vi "qc5psm2.vi"() -> ()   [LabVIEW 2020]
uses:
  <instrlib>/CAEN PSM/CAEN PSM.lvlib
panel:
  in  "Tab Control":enum32{"Page 1"}(tab)
  in  "Tab Control 2":enum32{"Page 1", "Page 2"}(tab)
  out "RDW":bool
  out "V monitor":dbl(graph)
  out "I monitor":dbl(graph)
  out "SHUT DOWN":bool
  out "COUNT VALUE":dynamicdata(graph)
  in  "count Time(sec)":dbl=60.0
  in  "Final Voltage":dbl=3250.0
  in  "V_step 1":dbl=200.0
  in  "VISA resource name":refnum<visa-resource-name>
  in  "Voltage ramp up (0 V/s)":u16 max=999
  in  "Voltage Max (0.0 V)":u16 max=9999
  in  "Board Address":i8 max=31
  in  "Vset_initial":dbl=100.0
  out "OVV 2":bool
  out "OVC 2":bool
  out "R calc":dbl
  out "Actual current level (Imon)":dbl
  out "Actual voltage level (Vmon)":dbl
  in  "START AGAIN":bool
  out "Channel Status Array":T1(array[cluster])
  in  "Channel (0)":u8=1
  in  "Req (Mohm)":dbl
  out "I set status":dbl
  in  "stop":bool
  in  "Middle Volt":dbl=3000.0
  in  "V step 2":dbl=100.0
  out "COUNT ON  TIMES":i16
  in  "device name":tag="Dev1"
  out "Counts":dbl
  out "time eclapsed":dbl format="%<%H:%M>t"
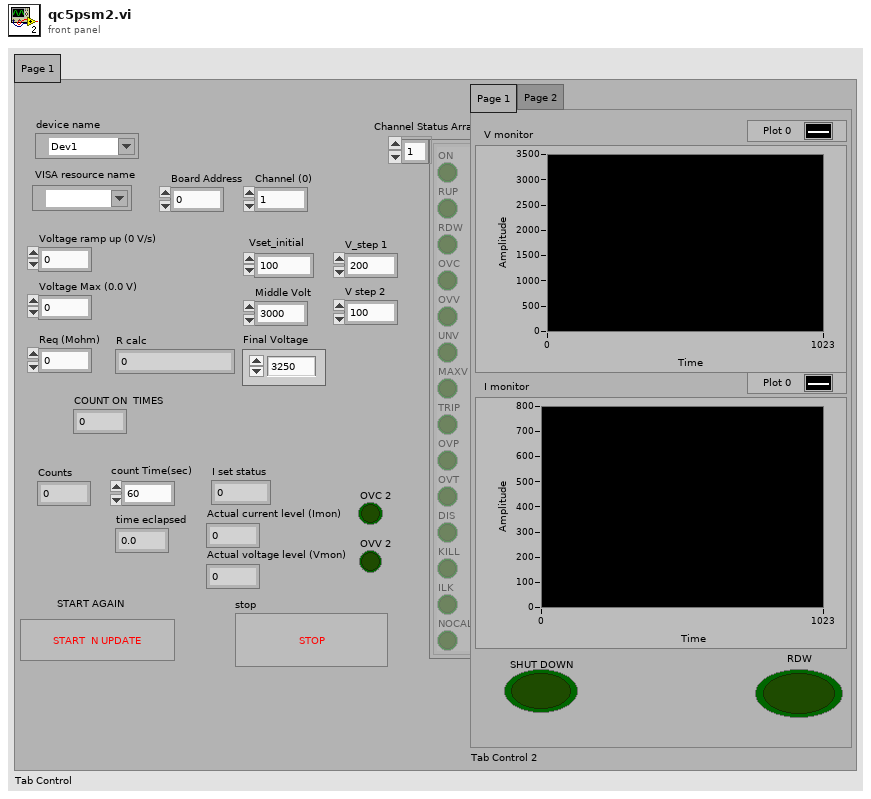
[diagram p1: front panel]
types:
  T1 = cluster{"ON":bool, "RUP":bool, "RDW":bool, "OVC":bool, "OVV":bool, "UNV":bool, "MAXV":bool, "TRIP":bool, "OVP":bool, "OVT":bool, "DIS":bool, "KILL":bool, "ILK":bool, "NOCAL":bool}[]
  T2 = cluster{"Baud Rate":u32, "Parity":enum16{"None", "Odd", "Even", "Mark", "Space"}, "Data Bits":u16, "Stop Bits":u16, "Flow Control":u16}
  T3 = typedef "CAEN PSM.lvlib/BoardHandle.ctl" = cluster{"VISA resource name":refnum<visa-resource-name>, "Board address":i8, "NChannels":u8}
  T4 = cluster{"ON":bool, "RUP":bool, "RDW":bool, "OVC":bool, "OVV":bool, "UNV":bool, "MAXV":bool, "TRIP":bool, "OVP":bool, "OVT":bool, "DIS":bool, "KILL":bool, "ILK":bool, "NOCAL":bool}
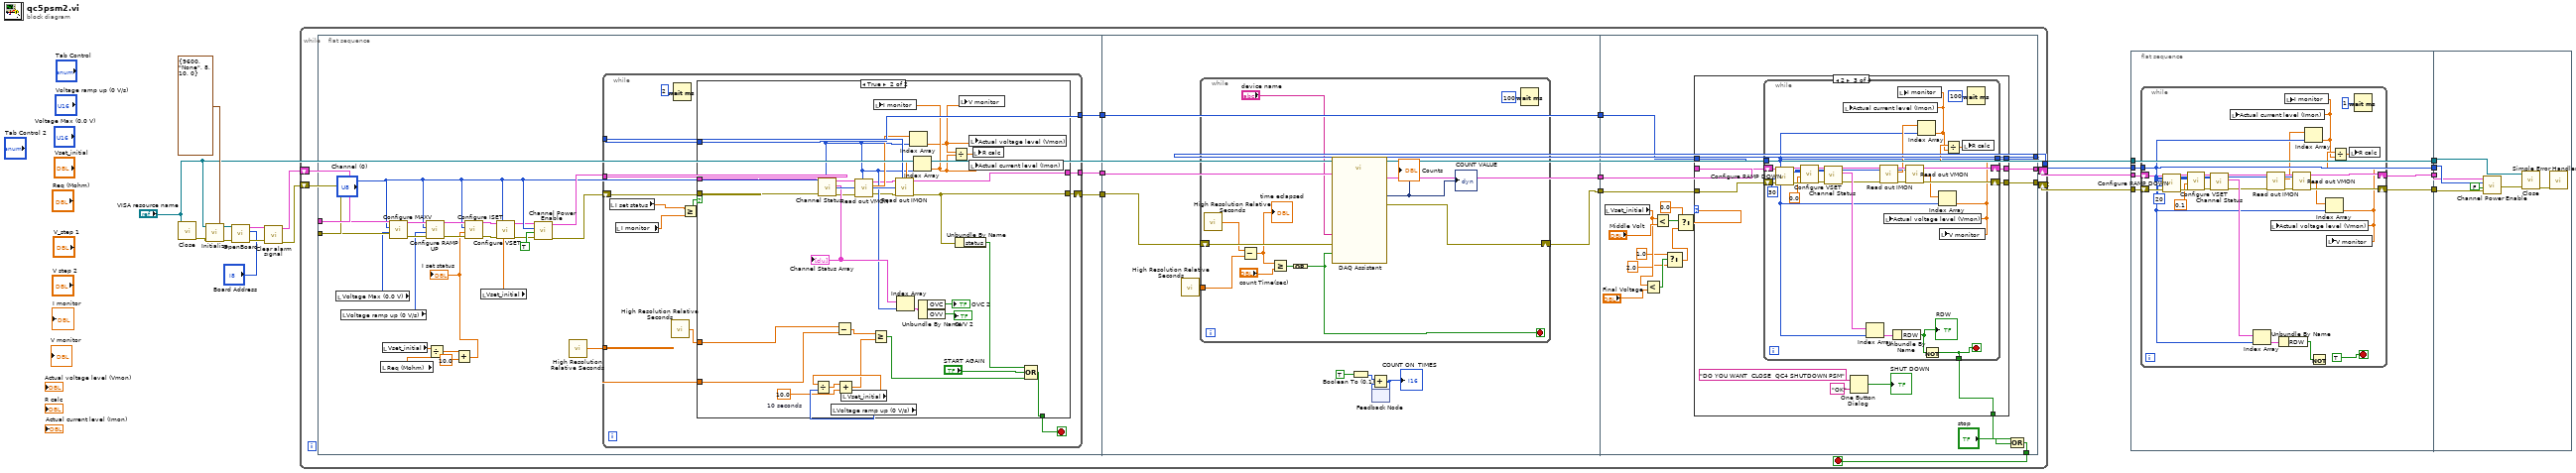
[diagram p0: block diagram]
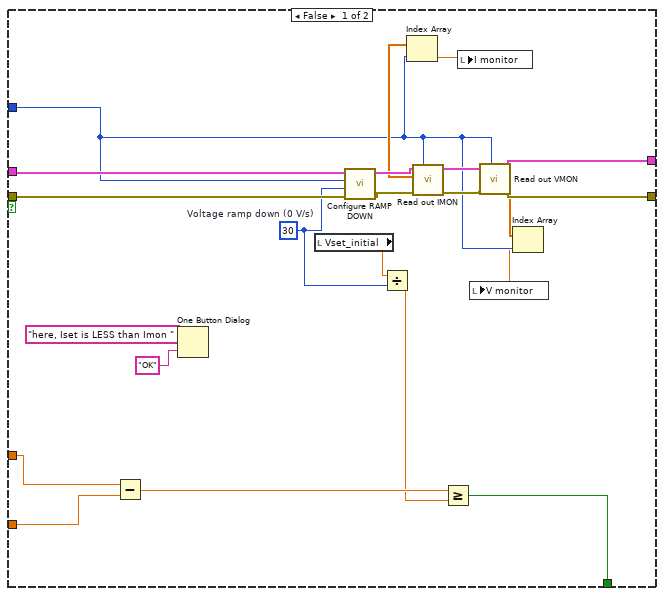
[diagram p2: hidden frame]
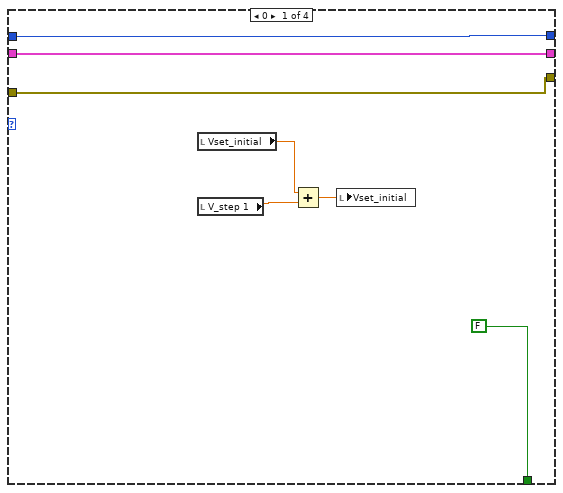
[diagram p3: hidden frame]
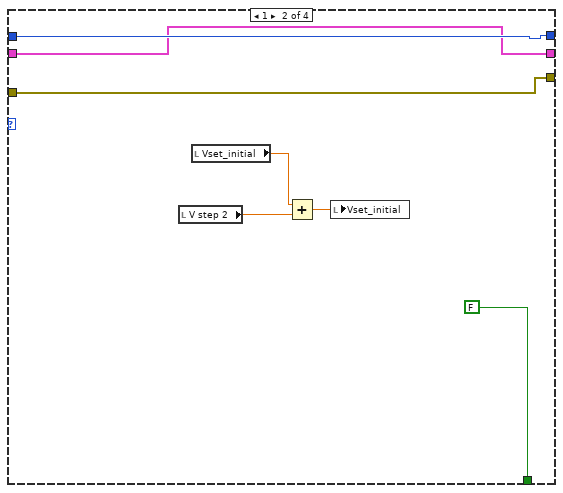
[diagram p4: hidden frame]
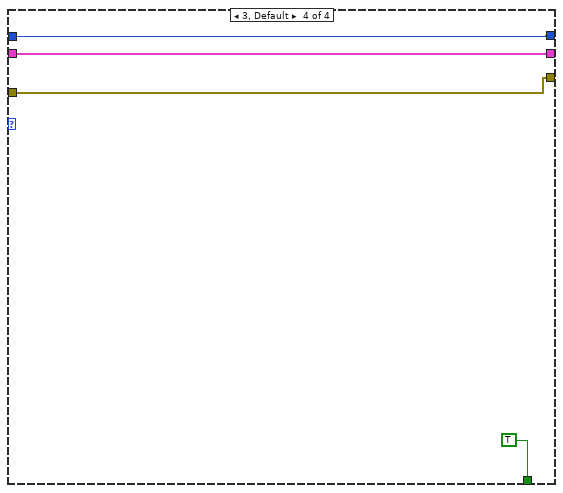
[diagram p5: hidden frame]
diagram:
  n1 = call <instrlib>:"Close.vi"("VISA resource name"="VISA resource name") -> ("error out"=w8:errorcluster)  [unwired: 10 in]
  n2 = call <instrlib>:"Initialize.vi"("Serial Configuration"=T2 {"Baud Rate"=9600, "Parity"=enum."None", "Data Bits"=8, "Stop Bits"=10, "Flow Control"=0}, "error in (no error)"=w8, "VISA resource name"="VISA resource name") -> ("error out"=w7:errorcluster, "VISA resource name out"=w16:refnum<visa-resource-name>)  [unwired: 7 in]
  n3 = call <instrlib>:"OpenBoard.vi"("error in (no error)"=w7, "Board Address"="Board Address", "VISA resource name"=w16) -> ("error out"=w14:errorcluster, "BoardHandle"=w15:T3)  [unwired: 7 in]
  n4 = call <instrlib>:"Clear alarm signal.vi"("error in (no error)"=w14, "BoardHandle"=w15) -> ("error out"=w9:errorcluster, "BoardHandle out"=w10:T3)  [unwired: 8 in]
  n5 = while {
    tunnel: [w29] -> w11
    shift-right: [w26] -> w6
    shift-left: w10 -> [w28]
    shift-right: [w18] -> w5
    shift-left: w9 -> [w27]
    stop <- w25 stop-if-true
    n6 = flat-sequence {
      tunnel: w28 -> [w53]
      tunnel: w27 -> [w52]
      tunnel: [w54] -> w24
      tunnel: [w33] -> w22
      tunnel: [w32] -> w20
      tunnel: w24 -> [w128]
      tunnel: [w128] -> w23
      tunnel: w22 -> [w127]
      tunnel: [w127] -> w21
      tunnel: w20 -> [w126]
      tunnel: [w125] -> w19
      tunnel: [w141] -> w18
      tunnel: [w140] -> w26
      tunnel: [w144] -> w29
      tunnel: w23 -> [w145]
      tunnel: w21 -> [w143]
      tunnel: w19 -> [w142]
      tunnel: [w147] -> w25
      frame #0 {
        n7 = local read "Voltage Max (0.0 V)"() -> (w48:u16)
        n8 = local read "Voltage ramp up (0 V/s)"() -> (w47:u16)
        n9 = local read "Req (Mohm)"() -> (w37:dbl)
        n10 = local read "Vset_initial"() -> (w38:dbl)
        n11 = call <instrlib>:"Configure MAXV.vi"("error in (no error)"=w52, "Voltage Max (0.0 V)"=w48, "Channel (0)"="Channel (0)", "BoardHandle"=w53) -> ("error out"=w49:errorcluster, "BoardHandle out"=w50:T3)  [unwired: 6 in]
        n12 = call <instrlib>:"Configure RAMP UP.vi"("error in (no error)"=w49, "Voltage ramp up (0 V/s)"=w47, "Channel (0)"="Channel (0)", "BoardHandle"=w50) -> ("error out"=w43:errorcluster, "BoardHandle out"=w45:T3)  [unwired: 6 in]
        n13 = Divide(x=w38, y=w37) -> (x/y=w40:dbl)
        n14 = Add(x=w40, y=10.0) -> (x+y=w30:dbl)
        "I set status" <- w30
        n15 = call <instrlib>:"Configure ISET.vi"("error in (no error)"=w43, "Current Limit (0.00 uA)"=w30, "Channel (0)"="Channel (0)", "BoardHandle"=w45) -> ("error out"=w42:errorcluster, "BoardHandle out"=w44:T3)  [unwired: 6 in]
        n16 = local read "Vset_initial"() -> (w41:dbl)
        n17 = call <instrlib>:"Configure VSET.vi"("error in (no error)"=w42, "Voltage Level (0.0 V)"=w41, "Channel (0)"="Channel (0)", "BoardHandle"=w44) -> ("error out"=w35:errorcluster, "BoardHandle out"=w34:T3)  [unwired: 6 in]
        n18 = call <instrlib>:"Channel Power Enable.vi"("error in (no error)"=w35, "Enable (OFF)"=TRUE, "Channel (0)"="Channel (0)", "BoardHandle"=w34) -> ("error out"=w51:errorcluster, "BoardHandle out"=w55:T3)  [unwired: 6 in]
        n19 = call <vilib>:"High Resolution Relative Seconds.vi"() -> ("relative seconds"=w31:dbl)
        n20 = while {
          shift-right: [w63] -> w32
          shift-left: w51 -> [w64]
          tunnel: [w62] -> w33
          tunnel: [w67] -> w54
          tunnel: w55 -> [w65]
          tunnel: "Channel (0)" -> [w67]
          tunnel: w31 -> [w60]
          stop <- w59 stop-if-true
          n21 = local read "I set status"() -> (w58:dbl)
          n22 = local read "I monitor"() -> (w56:dbl)
          n23 = call <vilib>:"High Resolution Relative Seconds.vi"() -> ("relative seconds"=w57:dbl)
          n24 = Wait (ms)(milliseconds to wait=u32 2) -> ()  [unwired: 1 out]
          n25 = Greater Or Equal?(x=w58, y=w56) -> (x >= y?=w61:bool)
          n26 = case shown="True" w61 {
            tunnel: w67 -> [w73 w113]
            tunnel: w65 -> [w89 w112]
            tunnel: w64 -> [w88 w111]
            tunnel: [w76 w110] -> w63
            tunnel: [w77 w109] -> w62
            tunnel: w60 -> [w87 w104]
            tunnel: [w82 w99] -> w59
            tunnel: w57 -> [w68 w90]
            frame False {
              w84 = u16 30  # Voltage ramp down (0 V/s)
              n27 = Subtract(x=w68, y=w87) -> (x-y=w86:dbl)
              n28 = One Button Dialog(message="here, Iset is LESS than Imon ", button name ("OK")="OK") -> ()  [unwired: 1 out]
              n29 = local read "Vset_initial"() -> (w85:dbl)
              n30 = call <instrlib>:"Configure RAMP DOWN.vi"("error in (no error)"=w88, "Voltage ramp down (0 V/s)"=w84, "Channel (0)"=w73, "BoardHandle"=w89) -> ("error out"=w80:errorcluster, "BoardHandle out"=w81:T3)  [unwired: 6 in]
              n31 = Divide(x=w85, y=w84) -> (x/y=w83:dbl)
              n32 = call <instrlib>:"Read out IMON.vi"("Channel"=w73, "error in (no error)"=w80, "BoardHandle"=w81) -> ("error out"=w78:errorcluster, "IMon values (uA)"=w75:dbl[], "BoardHandle out"=w79:T3)  [unwired: 5 in, 1 out]
              n33 = Index Array(array=w75, index=w73) -> (element=w70:dbl)
              n34 = Greater Or Equal?(x=w86, y=w83) -> (x >= y?=w82:bool)
              n35 = local write "I monitor"(w70) -> ()
              n36 = call <instrlib>:"Read out VMON.vi"("Channel"=w73, "error in (no error)"=w78, "BoardHandle"=w79) -> ("error out"=w76:errorcluster, "VMon values (V)"=w74:dbl[], "BoardHandle out"=w77:T3)  [unwired: 6 in]
              n37 = Index Array(array=w74, index=w73) -> (element=w69:dbl)
              n38 = local write "V monitor"(w69) -> ()
            }
            frame True {
              w95 = 10.0  # 10 seconds
              n39 = call <instrlib>:"Channel Status.vi"("Channel"=w113, "error in (no error)"=w111, "BoardHandle"=w112) -> ("error out"=w107:errorcluster, "Channel Status Array"=w118:T1, "BoardHandle out"=w108:T3)  [unwired: 5 in, 1 out]
              "Channel Status Array" <- w118
              n40 = local read "Voltage ramp up (0 V/s)"() -> (w97:u16)
              n41 = Subtract(x=w90, y=w104) -> (x-y=w101:dbl)
              n42 = local read "Vset_initial"() -> (w98:dbl)
              n43 = Divide(x=w98, y=w97) -> (x/y=w96:dbl)
              n44 = Add(x=w96, y=w95) -> (x+y=w94:dbl)
              n45 = call <instrlib>:"Read out VMON.vi"("Channel"=w113, "error in (no error)"=w107, "BoardHandle"=w108) -> ("error out"=w105:errorcluster, "VMon values (V)"=w119:dbl[], "BoardHandle out"=w106:T3)  [unwired: 6 in]
              n46 = Greater Or Equal?(x=w101, y=w94) -> (x >= y?=w103:bool)
              n47 = call <instrlib>:"Read out IMON.vi"("Channel"=w113, "error in (no error)"=w105, "BoardHandle"=w106) -> ("error out"=w110:errorcluster, "IMon values (uA)"=w114:dbl[], "BoardHandle out"=w109:T3)  [unwired: 5 in, 1 out]
              n48 = Index Array(array=w118, index=w113) -> (element=w117:T4)
              n49 = Index Array(array=w119, index=w113) -> (element=w91:dbl)
              n50 = Index Array(array=w114, index=w113) -> (element=w92:dbl)
              n51 = local write "I monitor"(w92) -> ()
              n52 = Unbundle By Name(w117) -> ("OVC"=→"OVC 2":bool, "OVV"=→"OVV 2":bool)
              n53 = Divide(x=w91, y=w92) -> (x/y=w93:dbl)
              n54 = Unbundle By Name(w110) -> ("status"=w100:bool)
              n55 = local write "V monitor"(w91) -> ()
              n56 = local write "Actual voltage level (Vmon)"(w91) -> ()
              n57 = local write "Actual current level (Imon)"(w92) -> ()
              n58 = local write "R calc"(w93) -> ()
              n59 = Compound Arithmetic op=OR(w100, "START AGAIN", w103) -> (w99:bool)
            }
          }
        }
      }
      frame #1 {
        n60 = call <vilib>:"High Resolution Relative Seconds.vi"() -> ("relative seconds"=w124:dbl)
        n61 = while {
          shift-right: [w138] -> w125
          shift-left: w126 -> [w139]
          tunnel: w124 -> [w133]
          stop <- w130 stop-if-true
          n62 = call <vilib>:"High Resolution Relative Seconds.vi"() -> ("relative seconds"=w135:dbl)
          n63 = Subtract(x=w135, y=w133) -> (x-y=w136:dbl)
          "time eclapsed" <- w136
          n64 = Greater Or Equal?(x=w136, y="count Time(sec)") -> (x >= y?=w134:bool)
          n65 = Compound Arithmetic op=OR(w134) -> (w130:bool)
          n66 = call "DAQ Assistant"("error in"=w139, "stop (F)"=w130, "device name"="device name") -> ("data"=→"Counts" →"COUNT VALUE":dynamicdata, "error out"=w138:errorcluster)  [unwired: 13 in, 2 out]
          n67 = Wait (ms)(milliseconds to wait=u32 100) -> ()  [unwired: 1 out]
        }
        n68 = Boolean To (0,1)(Boolean=TRUE) -> (0, 1=w123:i16)
        n69 = feedback #1() -> (w121:i16)  [unwired: 1 in]
        n70 = Add(x=w123, y=w121) -> (x+y=w122:i16)
        "COUNT ON  TIMES" <- w122
        n71 = feedback-in #1(w122) -> ()
      }
      frame #2 {
        n72 = local read "Vset_initial"() -> (w152:dbl)
        n73 = Less?(x=w152, y="Final Voltage") -> (x < y?=w155:bool)
        n74 = Less?(x=w152, y="Middle Volt") -> (x < y?=w157:bool)
        n75 = Select(t=1.0, s=w155, f=2.0) -> (s? t:f=w153:dbl)
        n76 = Select(t=0.0, s=w157, f=w153) -> (s? t:f=w158:dbl)
        n77 = case shown="2" w158 {
          tunnel: [FALSE FALSE w176 TRUE] -> w146
          tunnel: w145 -> [w161 w168 w182 w209]
          tunnel: [w161 w168 w181 w209] -> w144
          tunnel: w143 -> [w160 w167 w180 w208]
          tunnel: w142 -> [w159 w166 w179 w207]
          tunnel: [w159 w166 w177 w207] -> w141
          tunnel: [w160 w167 w178 w208] -> w140
          frame 0 {
            n78 = local read "Vset_initial"() -> (w165:dbl)
            n79 = local read "V_step 1"() -> (w163:dbl)
            n80 = Add(x=w165, y=w163) -> (x+y=w164:dbl)
            n81 = local write "Vset_initial"(w164) -> ()
          }
          frame 1 {
            n82 = local read "V step 2"() -> (w170:dbl)
            n83 = local read "Vset_initial"() -> (w172:dbl)
            n84 = Add(x=w172, y=w170) -> (x+y=w171:dbl)
            n85 = local write "Vset_initial"(w171) -> ()
          }
          frame 2 {
            n86 = while {
              tunnel: w182 -> [w184]
              shift-right: [w204] -> w178
              shift-left: w180 -> [w206]
              shift-right: [w203] -> w177
              shift-left: w179 -> [w205]
              tunnel: [w184] -> w181
              tunnel: [w183] -> w176
              stop <- w183 stop-if-true
              n87 = call <instrlib>:"Configure RAMP DOWN.vi"("error in (no error)"=w205, "Voltage ramp down (0 V/s)"=u16 30, "Channel (0)"=w184, "BoardHandle"=w206) -> ("error out"=w199:errorcluster, "BoardHandle out"=w200:T3)  [unwired: 6 in]
              n88 = call <instrlib>:"Configure VSET.vi"("error in (no error)"=w199, "Voltage Level (0.0 V)"=0.0, "Channel (0)"=w184, "BoardHandle"=w200) -> ("error out"=w196:errorcluster, "BoardHandle out"=w197:T3)  [unwired: 6 in]
              n89 = call <instrlib>:"Channel Status.vi"("Channel"=w184, "error in (no error)"=w196, "BoardHandle"=w197) -> ("error out"=w191:errorcluster, "Channel Status Array"=w195:T1, "BoardHandle out"=w190:T3)  [unwired: 5 in, 1 out]
              n90 = Index Array(array=w195, index=w184) -> (element=w194:T4)
              n91 = call <instrlib>:"Read out IMON.vi"("Channel"=w184, "BoardHandle"=w190) -> ("IMon values (uA)"=w188:dbl[], "BoardHandle out"=w189:T3)  [unwired: 6 in, 2 out]
              n92 = Unbundle By Name(w194) -> ("RDW"=w193:bool)
              "RDW" <- w193
              n93 = call <instrlib>:"Read out VMON.vi"("Channel"=w184, "error in (no error)"=w191, "BoardHandle"=w189) -> ("error out"=w203:errorcluster, "VMon values (V)"=w201:dbl[], "BoardHandle out"=w204:T3)  [unwired: 6 in]
              n94 = Index Array(array=w188, index=w184) -> (element=w185:dbl)
              n95 = local write "Actual current level (Imon)"(w185) -> ()
              n96 = local write "I monitor"(w185) -> ()
              n97 = Not(x=w193) -> (.not. x?=w183:bool)
              n98 = Index Array(array=w201, index=w184) -> (element=w186:dbl)
              n99 = local write "Actual voltage level (Vmon)"(w186) -> ()
              n100 = local write "V monitor"(w186) -> ()
              n101 = Divide(x=w186, y=w185) -> (x/y=w187:dbl)
              n102 = local write "R calc"(w187) -> ()
              n103 = Wait (ms)(milliseconds to wait=u32 100) -> ()  [unwired: 1 out]
            }
            n104 = One Button Dialog(message="DO YOU WANT  CLOSE  QC4 SHUTDOWN PSM", button name ("OK")="OK") -> (true=→"SHUT DOWN":bool)
          }
          frame 3, Default {
          }
        }
        n105 = Compound Arithmetic op=OR(w146, "stop") -> (w147:bool)
      }
    }
  }
  n106 = flat-sequence {
    tunnel: w5 -> [w214]
    tunnel: w6 -> [w215]
    tunnel: w11 -> [w211]
    tunnel: "VISA resource name" -> [w216]
    tunnel: [w216] -> w4
    tunnel: [w211] -> w3
    tunnel: [w213] -> w2
    tunnel: [w212] -> w1
    tunnel: w4 -> [w245]
    tunnel: w3 -> [w243]
    tunnel: w2 -> [w242]
    tunnel: w1 -> [w241]
    frame #0 {
      n107 = while {
        tunnel: w211 -> [w228]
        shift-right: [w238] -> w213
        shift-left: w215 -> [w240]
        shift-right: [w237] -> w212
        shift-left: w214 -> [w239]
        stop <- TRUE stop-if-true
        n108 = call <instrlib>:"Configure RAMP DOWN.vi"("error in (no error)"=w239, "Voltage ramp down (0 V/s)"=u16 20, "Channel (0)"=w228, "BoardHandle"=w240) -> ("error out"=w233:errorcluster, "BoardHandle out"=w234:T3)  [unwired: 6 in]
        n109 = call <instrlib>:"Configure VSET.vi"("error in (no error)"=w233, "Voltage Level (0.0 V)"=0.1, "Channel (0)"=w228, "BoardHandle"=w234) -> ("error out"=w230:errorcluster, "BoardHandle out"=w231:T3)  [unwired: 6 in]
        n110 = call <instrlib>:"Channel Status.vi"("Channel"=w228, "error in (no error)"=w230, "BoardHandle"=w231) -> ("error out"=w224:errorcluster, "Channel Status Array"=w229:T1, "BoardHandle out"=w223:T3)  [unwired: 5 in, 1 out]
        n111 = Index Array(array=w229, index=w228) -> (element=w227:T4)
        n112 = call <instrlib>:"Read out IMON.vi"("Channel"=w228, "BoardHandle"=w223) -> ("IMon values (uA)"=w221:dbl[], "BoardHandle out"=w222:T3)  [unwired: 6 in, 2 out]
        n113 = Unbundle By Name(w227) -> ("RDW"=w226:bool)
        n114 = call <instrlib>:"Read out VMON.vi"("Channel"=w228, "error in (no error)"=w224, "BoardHandle"=w222) -> ("error out"=w237:errorcluster, "VMon values (V)"=w235:dbl[], "BoardHandle out"=w238:T3)  [unwired: 6 in]
        n115 = Index Array(array=w221, index=w228) -> (element=w218:dbl)
        n116 = local write "Actual current level (Imon)"(w218) -> ()
        n117 = local write "I monitor"(w218) -> ()
        n118 = Not(x=w226) -> ()  [unwired: 1 out]
        n119 = Index Array(array=w235, index=w228) -> (element=w219:dbl)
        n120 = local write "Actual voltage level (Vmon)"(w219) -> ()
        n121 = local write "V monitor"(w219) -> ()
        n122 = Divide(x=w219, y=w218) -> (x/y=w220:dbl)
        n123 = local write "R calc"(w220) -> ()
        n124 = Wait (ms)(milliseconds to wait=u32 1) -> ()  [unwired: 1 out]
      }
    }
    frame #1 {
      n125 = call <instrlib>:"Channel Power Enable.vi"("error in (no error)"=w241, "Enable (OFF)"=FALSE, "Channel (0)"=w243, "BoardHandle"=w242) -> ("error out"=w247:errorcluster)  [unwired: 6 in, 1 out]
      n126 = call <instrlib>:"Close.vi"("error in (no error)"=w247, "VISA resource name"=w245) -> ("error out"=w246:errorcluster)  [unwired: 9 in]
      n127 = call <vilib>:"Simple Error Handler.vi"("error in (no error)"=w246) -> ()  [unwired: 4 in, 5 out]
    }
  }
